vi "Video Test.vi"(11 "VideoValue":dbl format="%.2f") -> (0 "error out":errorcluster, 3 "Latency (µs)":dbl format="%.2f")   [LabVIEW 2025]
doc: "Tests the video card installed on the motherboard. Returns a value indicating the response time of the video card."
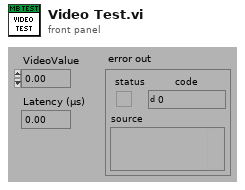
[diagram p1: front panel]
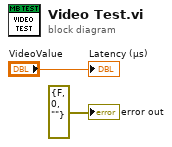
[diagram p0: block diagram]
diagram:
  "error out" <- errorcluster {"status"=FALSE, "code"=0, "source"=""} ("error out")
  "Latency (µs)" <- "VideoValue"
